vi "Fusion Multicast Receiver.vi"() -> ()   [LabVIEW 2015]
doc: "Creates a read-only UDP multicast session and receives data on the specified port."
uses:
  <vilib>/Utility/tcp.llb/UDP Multicast Read-Only Open.vi
panel:
  out "Sensor Fusion Data":dbl(graph)
  in  "Stop":bool
  # "Overview: Demonstrates the use of the UDP functions to connect to a UDP multicast session and receive data.\nInstructions:\n1. Ensure UDP Multicast - Sender.vi is already running.\n2. Run the VI.\n3. Click Stop to stop the VI."
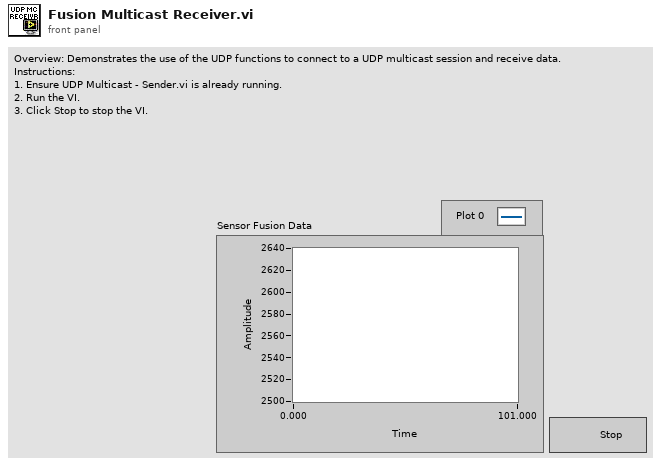
[diagram p1: front panel]
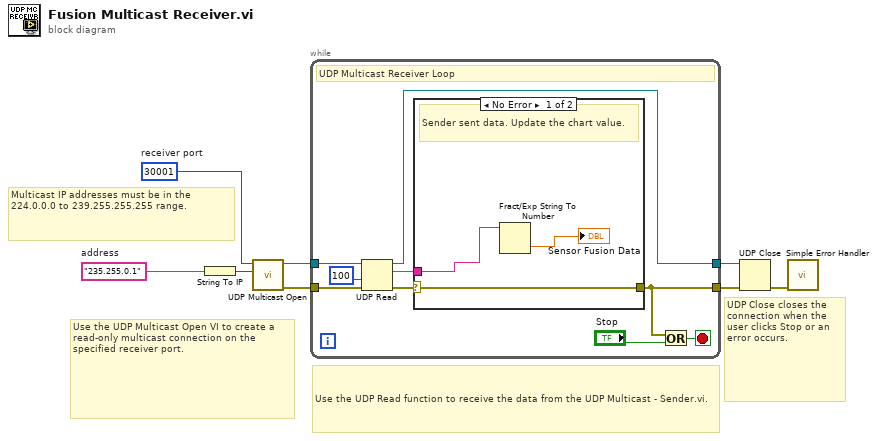
[diagram p0: block diagram]
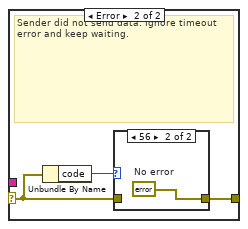
[diagram p2: hidden frame]
diagram:
  w2 = u16 30001  # receiver port
  w7 = "235.255.0.1"  # address
  # "UDP Close closes the connection when the user clicks Stop or an error occurs."
  # "Use the UDP Multicast Open VI to create a read-only multicast connection on the specified receiver port."
  # "Multicast IP addresses must be in the 224.0.0.0 to 239.255.255.255 range."
  # "Use the UDP Read function to receive the data from the UDP Multicast - Sender.vi."
  n1 = String To IP(1:w7) -> (0:w1:u32)
  n2 = call-poly <vilib>:"UDP Multicast Open.vi"("multicast addr"=w1, "port"=w2) -> ("error out"=w4:errorcluster, "connection ID"=w3:refnum<k16>)  [unwired: 7 in, 1 out]
  n3 = while {
    tunnel: w3 -> [w17]
    tunnel: [w9] -> w8
    tunnel: w4 -> [w14]
    tunnel: [w10] -> w5
    stop <- w15 stop-if-true
    # "UDP Multicast Receiver Loop"
    n4 = UDP Read(connection ID=w17, timeout ms (25000)=100, 8:w14) -> (data out=w12:string, error out=w11:errorcluster, 3:w9:refnum<k16>)  [unwired: 3 out]
    n5 = case shown="No Error" w11 {
      selector: w11 -> [w20 w22]
      tunnel: w12 -> [w19 _]
      tunnel: [w20 w21] -> w10
      frame No Error {
        # "Sender sent data. Update the chart value."
        n6 = Fract/Exp String To Number(string=w19) -> (number=→"Sensor Fusion Data":dbl)  [unwired: 3 in, 1 out]
      }
      frame Error {
        # "Sender did not send data. Ignore timeout error and keep waiting."
        n7 = Unbundle By Name(w22) -> ("code"=w23:i32)
        n8 = case shown="56" w23 {
          tunnel: w22 -> [w24 _]
          tunnel: [w24 w25] -> w21
          frame Default {
          }
          frame 56 {
            w25 = errorcluster {"status"=FALSE, "code"=0, "source"=""}  # No error
          }
        }
      }
    }
    n9 = Or(x=w10, y="Stop") -> (x .or. y?=w15:bool)
  }
  n10 = UDP Close(connection ID=w8, 8:w5) -> (error out=w6:errorcluster)  [unwired: 1 out]
  n11 = call <vilib>:"Simple Error Handler.vi"("error in (no error)"=w6) -> ()  [unwired: 1 in, 8 out]
